vi "RGB LED Write.vi"(8 "Error In":errorcluster, 9 "Color":u32(colorbox), 10 "RGB LED Pins":u8[](array[numeric])=[3, 5, 6], 11 "ChipKit Resource":T1={"COM Port"="", "Board Type"=enum."ChipKit uC32", "Connection Type"=enum."USB / Serial", "Baud Rate (115200)"=15, "Bytes Per Packet (15)"=15}) -> (0 "Error Out":errorcluster, 2 "RGB LED Pins":u8[](array[numeric]), 3 "ChipKit Resource":T1={"COM Port"="", "Board Type"=enum."ChipKit uC32", "Connection Type"=enum."USB / Serial", "Baud Rate (115200)"=15, "Bytes Per Packet (15)"=15})   [LabVIEW 2011, in "LabVIEW Interface for ChipKit.lvlib"]
doc: "Write color value to RGB LED. Arduino Configure RGB LED must be called to configure the RGB LED pins before calling this VI."
uses:
  LabVIEW Interface for ChipKit.lvlib
  Private/Type Defs/Board Type.ctl
  Private/Type Defs/Chipkit Resource.ctl
  Private/Type Defs/Connection Type.ctl
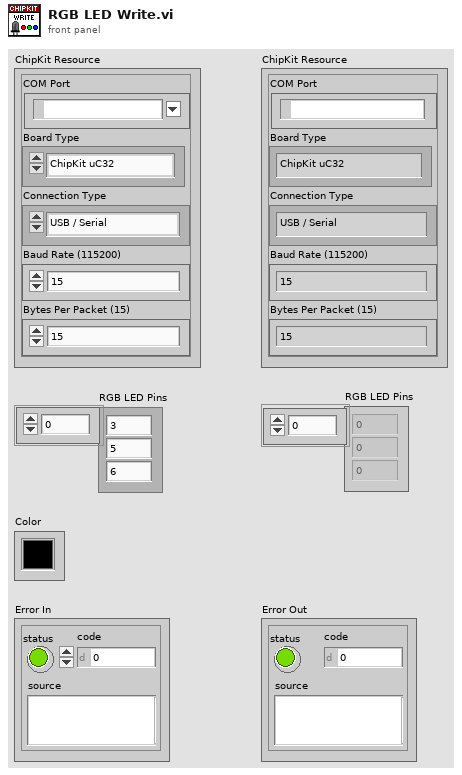
[diagram p1: front panel]
types:
  T1 = typedef "LabVIEW Interface for ChipKit.lvlib/Chipkit Resource.ctl" = cluster{"COM Port":refnum<visa-resource-name>, "Board Type":T2, "Connection Type":T3, "Baud Rate (115200)":u32, "Bytes Per Packet (15)":u32}
  T2 = typedef "LabVIEW Interface for ChipKit.lvlib/Board Type.ctl" = enum16{"ChipKit uC32", "ChipKit Uno32", "ChipKit Max32"}
  T3 = typedef "LabVIEW Interface for ChipKit.lvlib/Connection Type.ctl" = enum8{"USB / Serial", "XBEE", "BlueSmirf (Bluetooth)"}
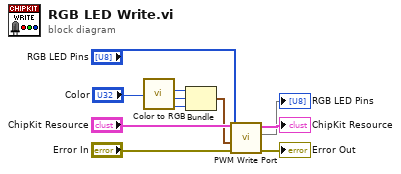
[diagram p0: block diagram]
diagram:
  n1 = call <vilib>:"Color to RGB.vi"("Color"="Color") -> ("R"=w6:u8, "G"=w5:u8, "B"=w4:u8)  [unwired: 1 out]
  n2 = Bundle("R"=w6, "G"=w5, "B"=w4) -> (w3:cluster{"R":u8, "G":u8, "B":u8})  [unwired: 1 in]
  n3 = call "PWM Write Port.vi"("Error In"="Error In", 9:w3, "Duty Cycles"="RGB LED Pins", "ChipKit Resource"="ChipKit Resource") -> ("Error Out"=→"Error Out":errorcluster, 2:→"RGB LED Pins", "ChipKit Resource"=→"ChipKit Resource":T1)  [unwired: 5 in]
